vi "RSNRPZ Get Scope Measurements Algorithm.vi"(8 "error in (no error)":errorcluster, 10 "Channel (1)":i32=1, 11 "VISA session":refnum<visa-resource-name> caption="VISA resource name") -> (0 "error out":errorcluster, 1 "Algorithm":i32, 3 "dup VISA session":refnum<visa-resource-name> caption="VISA resource name")   [LabVIEW 2010]
doc: "This VI queries selected algorithm for detecting the top and the base level of the pulsed signal.\n\nNote:\n1) This VI is only available for NRP-Z81.\n\nRemote-control command(s):\nSENS:TRAC:MEAS:ALG?"
uses:
  rsnrpz_32.dll
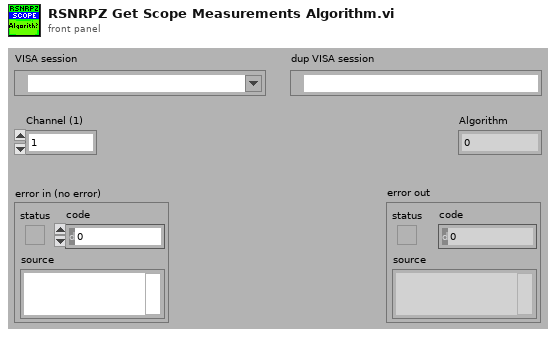
[diagram p1: front panel]
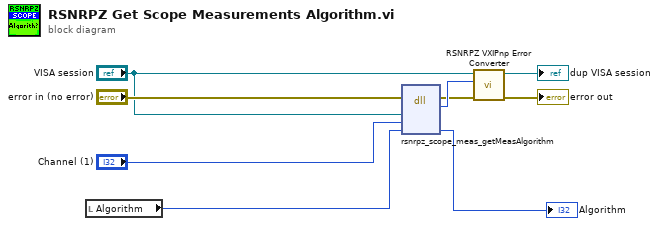
[diagram p0: block diagram]
diagram:
  n1 = local read "Algorithm"() -> (w7:i32)
  n2 = dll-call lib="rsnrpz_32.dll" fn="rsnrpz_scope_meas_getMeasAlgorithm"(error in="error in (no error)", "Instrument Handle"="VISA session", "Channel"="Channel (1)", "Algorithm"=w7) -> (error out=w5:errorcluster, "Status"=w9:i32, "Algorithm"=→"Algorithm":i32)  [unwired: 4 in, 1 out]
  n3 = call <instrlib>:"RSNRPZ VXIPnp Error Converter.vi"("error in"=w5, "VXIPnp error code"=w9, "VISA session"="VISA session") -> ("error out"=→"error out":errorcluster, "dup VISA session"=→"dup VISA session":refnum<visa-resource-name>)  [unwired: 7 in]
